vi "read_sub_sampling.vi"(8 "error in (no error)":errorcluster, 11 "LatentDirichletAllocation in":refnum<class "LatentDirichletAllocation.lvclass">) -> (0 "error out":errorcluster, 2 "sub_sampling":bool, 3 "LatentDirichletAllocation out":refnum<class "LatentDirichletAllocation.lvclass">)   [LabVIEW 2020, in "LatentDirichletAllocation.lvclass"]
uses:
  LatentDirichletAllocation.lvclass
  LatentDirichletAllocation.lvclass/LatentDirichletAllocation.ctl
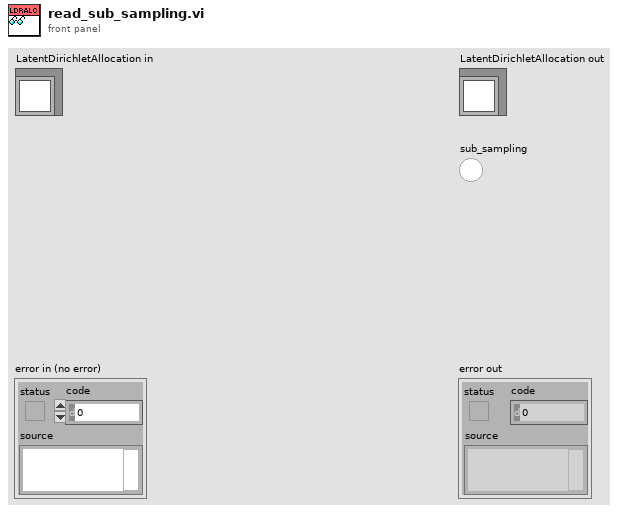
[diagram p1: front panel]
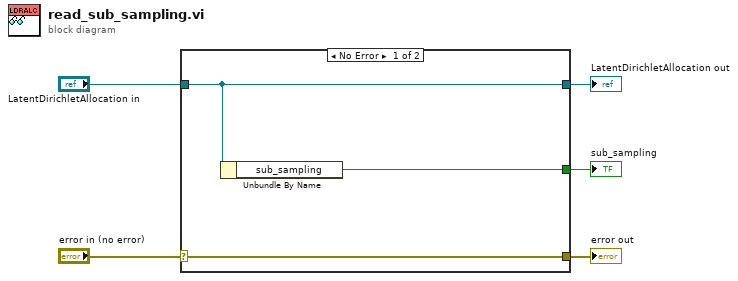
[diagram p0: block diagram]
diagram:
  n1 = case shown="No Error" "error in (no error)" {
    selector: "error in (no error)" -> [w8 w9]
    tunnel: [w8 w9] -> w4
    tunnel: [w7 w10] -> w2
    tunnel: "LatentDirichletAllocation in" -> [w7 w10]
    tunnel: [w6 _] -> w1
    frame No Error {
      n2 = Unbundle By Name(w7) -> ("sub_sampling"=w6:bool)
    }
    frame Error {
    }
  }
  "error out" <- w4
  "LatentDirichletAllocation out" <- w2
  "sub_sampling" <- w1
